vi "Pockels Cal-Event handler-Use sel file.vi"(11 "Cal files listbox":refnum<vi>) -> (0 "error out":errorcluster)   [LabVIEW 2017]
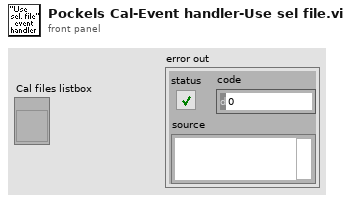
[diagram p1: front panel]
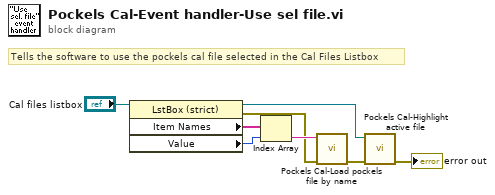
[diagram p0: block diagram]
diagram:
  # "Tells the software to use the pockels cal file selected in the Cal Files Listbox"
  n1 = property on="Property Node" class="LstBox (strict)"(reference="Cal files listbox") -> (reference out=w1:refnum<vi>, error out=w4:errorcluster, "Item Names"=w5:string[], "Value"=w6:i32)  [unwired: 1 in]
  n2 = Index Array(array=w5, index=w6) -> (element=w8:string)
  n3 = call "Pockels Cal-Load pockels file by name.vi"("error in"=w4, "Pockels cal file name"=w8) -> ("error out"=w3:errorcluster)  [unwired: 8 in, 1 out]
  n4 = call "Pockels Cal-Highlight active file.vi"("error in (no error)"=w3, "ListBox in"=w1) -> ("error out"=→"error out":errorcluster)  [unwired: 9 in]
